vi "InsertRunner'sData.vi"(8 "error in":errorcluster, 11 "Runners Data":T1) -> (0 "error out":errorcluster, 2 "Canceled?":bool, 3 "Runners Data Out":T1)   [LabVIEW 2021]
doc: "This Vi generates new Runner's Data.\nCancelled? indicator equals true if it was cancelled."
uses:
  Controls/Runner's Data.ctl
panel:
  in  "Cancel Button":bool
  in  "OK Button":bool
  # "Share your data and click OK"
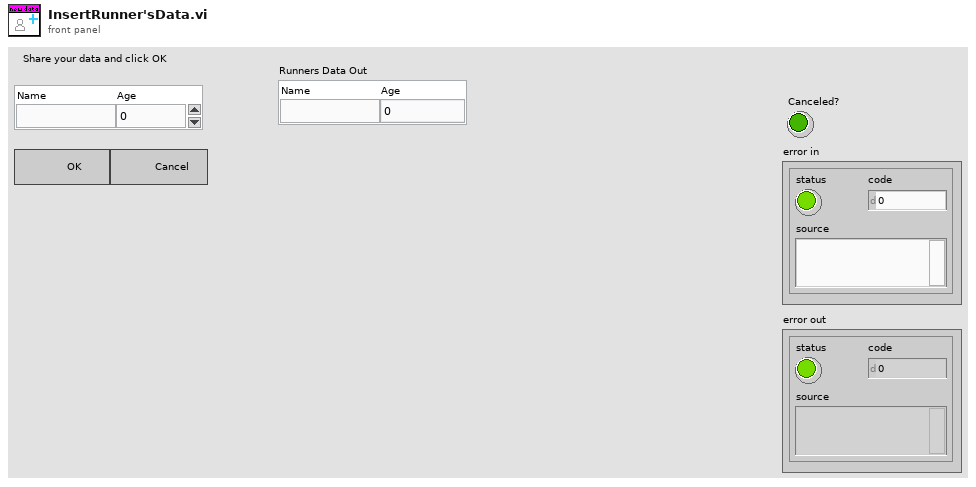
[diagram p1: front panel]
types:
  T1 = typedef "Runner's Data.ctl" = cluster{"Name":string, "Age":i32}
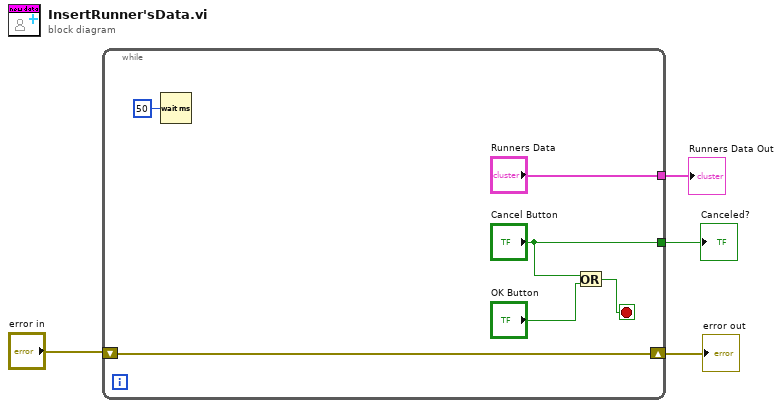
[diagram p0: block diagram]
diagram:
  n1 = while {
    shift-right: [w10] -> w3
    shift-left: "error in" -> [w10]
    tunnel: ["Runners Data"] -> w2
    tunnel: ["Cancel Button"] -> w1
    stop <- w9 stop-if-true
    n2 = Wait (ms)(milliseconds to wait=u32 50) -> ()  [unwired: 1 out]
    n3 = Or(x="Cancel Button", y="OK Button") -> (x .or. y?=w9:bool)
  }
  "error out" <- w3
  "Runners Data Out" <- w2
  "Canceled?" <- w1
